vi "Key Pressed.vi"(2 "1D array":T1(array[ring])) -> (12 "1":bool, 13 "3":bool, 15 "2":bool, 18 "4":bool)   [LabVIEW 2011]
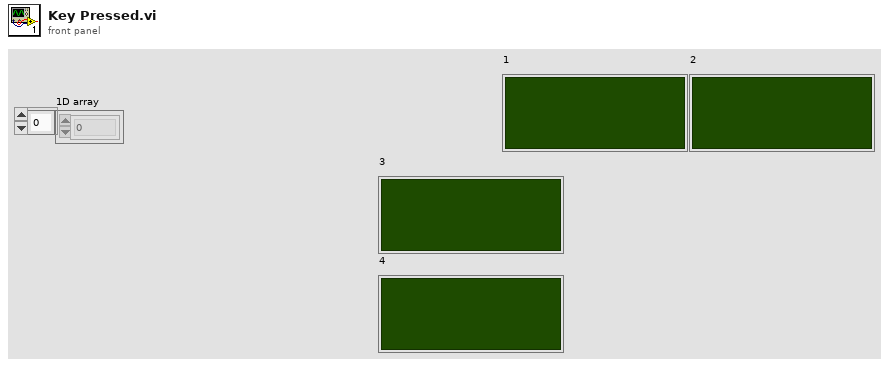
[diagram p1: front panel]
types:
  T1 = enum16{"0", "1", "2", "3", "4", "5", "6", "7", "8", "9", "A", "B", "C", "D", "E", "F", "G", "H", "I", "J", "K", "L", "M", "N", "O", "P", "Q", "R", "S", "T", "U", "V", "W", "X", "Y", "Z", "F1", "F2", "F3", "F4", "F5", "F6", "F7", "F8", "F9", "F10", "F11", "F12", "F13", "F14", "F15", "ADD", "BACK", "BACKSLASH", "CAPITAL", "COMMA", "DECIMAL", "DELETE", "DIVIDE", "DOWN", "END", "EQUALS", "ESCAPE", "GRAVE (`)", "HOME", "INSERT", "LBRACKET", "LCONTROL", "LEFT", "L ALT", "LSHIFT", "LWIN", "MINUS", "MULTIPLY", "NEXT", "NUMLOCK", "NUMPAD_0", "NUMPAD_1", "NUMPAD_2", "NUMPAD_3", "NUMPAD_4", "NUMPAD_5", "NUMPAD_6", "NUMPAD_7", "NUMPAD_8", "NUMPAD_9", "PAUSE", "PERIOD", "PRIOR (PG UP)", "RBRACKET", "RCONTROL", "RETURN", "RIGHT", "R ALT", "RSHIFT", "RWIN", "SCROLL", "SEMICOLON", "SLASH", "SPACE", "SUBTRACT", "TAB", "UP", "ENTER (num pad)", "' (quote)"}[]
  T2 = enum16{"0", "1", "2", "3", "4", "5", "6", "7", "8", "9", "A", "B", "C", "D", "E", "F", "G", "H", "I", "J", "K", "L", "M", "N", "O", "P", "Q", "R", "S", "T", "U", "V", "W", "X", "Y", "Z", "F1", "F2", "F3", "F4", "F5", "F6", "F7", "F8", "F9", "F10", "F11", "F12", "F13", "F14", "F15", "ADD", "BACK", "BACKSLASH", "CAPITAL", "COMMA", "DECIMAL", "DELETE", "DIVIDE", "DOWN", "END", "EQUALS", "ESCAPE", "GRAVE (`)", "HOME", "INSERT", "LBRACKET", "LCONTROL", "LEFT", "L ALT", "LSHIFT", "LWIN", "MINUS", "MULTIPLY", "NEXT", "NUMLOCK", "NUMPAD_0", "NUMPAD_1", "NUMPAD_2", "NUMPAD_3", "NUMPAD_4", "NUMPAD_5", "NUMPAD_6", "NUMPAD_7", "NUMPAD_8", "NUMPAD_9", "PAUSE", "PERIOD", "PRIOR (PG UP)", "RBRACKET", "RCONTROL", "RETURN", "RIGHT", "R ALT", "RSHIFT", "RWIN", "SCROLL", "SEMICOLON", "SLASH", "SPACE", "SUBTRACT", "TAB", "UP", "ENTER (num pad)", "' (quote)"}
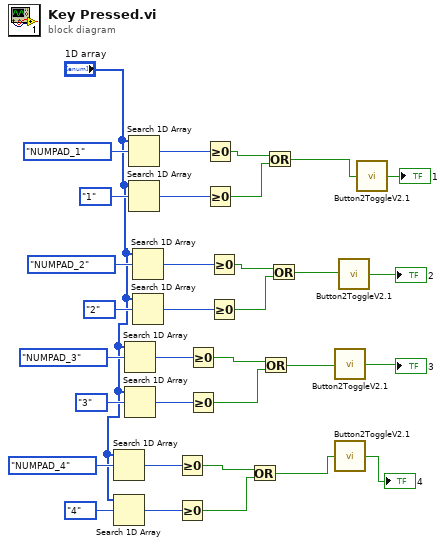
[diagram p0: block diagram]
diagram:
  n1 = Search 1D Array(1D array="1D array", element=T2."NUMPAD_4" ("keys pressed[0]")) -> (index of element=w10:i32)  [unwired: 1 in]
  n2 = Search 1D Array(1D array="1D array", element=T2."4" ("keys pressed[0]")) -> (index of element=w13:i32)  [unwired: 1 in]
  n3 = Search 1D Array(1D array="1D array", element=T2."NUMPAD_3" ("keys pressed[0]")) -> (index of element=w21:i32)  [unwired: 1 in]
  n4 = Search 1D Array(1D array="1D array", element=T2."3" ("keys pressed[0]")) -> (index of element=w18:i32)  [unwired: 1 in]
  n5 = Search 1D Array(1D array="1D array", element=T2."NUMPAD_1" ("keys pressed[0]")) -> (index of element=w33:i32)  [unwired: 1 in]
  n6 = Search 1D Array(1D array="1D array", element=T2."1" ("keys pressed[0]")) -> (index of element=w30:i32)  [unwired: 1 in]
  n7 = Search 1D Array(1D array="1D array", element=T2."NUMPAD_2" ("keys pressed[0]")) -> (index of element=w22:i32)  [unwired: 1 in]
  n8 = Search 1D Array(1D array="1D array", element=T2."2" ("keys pressed[0]")) -> (index of element=w25:i32)  [unwired: 1 in]
  n9 = Greater Or Equal To 0?(x=w10) -> (x >= 0?=w14:bool)
  n10 = Greater Or Equal To 0?(x=w13) -> (x >= 0?=w15:bool)
  n11 = Greater Or Equal To 0?(x=w21) -> (x >= 0?=w17:bool)
  n12 = Greater Or Equal To 0?(x=w18) -> (x >= 0?=w16:bool)
  n13 = Greater Or Equal To 0?(x=w33) -> (x >= 0?=w29:bool)
  n14 = Greater Or Equal To 0?(x=w30) -> (x >= 0?=w28:bool)
  n15 = Greater Or Equal To 0?(x=w22) -> (x >= 0?=w26:bool)
  n16 = Greater Or Equal To 0?(x=w25) -> (x >= 0?=w27:bool)
  n17 = Or(x=w14, y=w15) -> (x .or. y?=w6:bool)
  n18 = Or(x=w17, y=w16) -> (x .or. y?=w7:bool)
  n19 = Or(x=w29, y=w28) -> (x .or. y?=w9:bool)
  n20 = Or(x=w26, y=w27) -> (x .or. y?=w8:bool)
  n21 = call "Button2ToggleV2.1.vi"("a"=w7) -> ("Result(clone)"=→"3":bool)
  n22 = call "Button2ToggleV2.1.vi"("a"=w6) -> ("Result(clone)"=→"4":bool)
  n23 = call "Button2ToggleV2.1.vi"("a"=w8) -> ("Result(clone)"=→"2":bool)
  n24 = call "Button2ToggleV2.1.vi"("a"=w9) -> ("Result(clone)"=→"1":bool)
